vi "Acquire.vi"(6 "Count In":i32, 8 "error in (no error)":errorcluster, 9 "Data Queue":refnum<queue>, 10 "APD Data Notifier":refnum<notifier>, 11 "HW Resources In":T1={"Data Source"=0, "Counter Configuration"={"DAQmx Task"="", "Counter(s)"="Dev2/ctr0", "samples per readout"=100}, "ADC Configuration"={"DAQmx Task"="", "Channel(s)"="Dev2/ctr0", "samples per readout"=100, "Sample Rate (s/s)"=100, "Max Voltage"=100.0, "Min Voltage"=100.0}} {"Data Source" items=["Counter", "ADC"]}) -> (0 "error out":errorcluster, 3 "HW Resources Out":T1={"Data Source"=0, "Counter Configuration"={"DAQmx Task"="", "Counter(s)"="Dev2/ctr0", "samples per readout"=100}, "ADC Configuration"={"DAQmx Task"="", "Channel(s)"="Dev2/ctr0", "samples per readout"=100, "Sample Rate (s/s)"=100, "Max Voltage"=100.0, "Min Voltage"=100.0}} {"Data Source" items=["Counter", "ADC"]}, 4 "Cout Out":i32)   [LabVIEW 2013, in "Acquisition.lvlib"]
doc: "Perform the acquisition. Replace the contents of this diagram with calls to acquisition hardware."
uses:
  Acquisition.lvlib
  Hardware Configuration.ctl
  Counter Configuration.ctl
  ADC/ADC Configuration.ctl
  APD Notifier Cluster.ctl
  <vilib>/DAQmx/read.llb/DAQmx Read (Counter 1D DBL 1Chan NSamp).vi
  <vilib>/DAQmx/read.llb/DAQmx Read (Analog 1D Wfm NChan NSamp).vi
  <resource>/objmgr/daqmx.rc
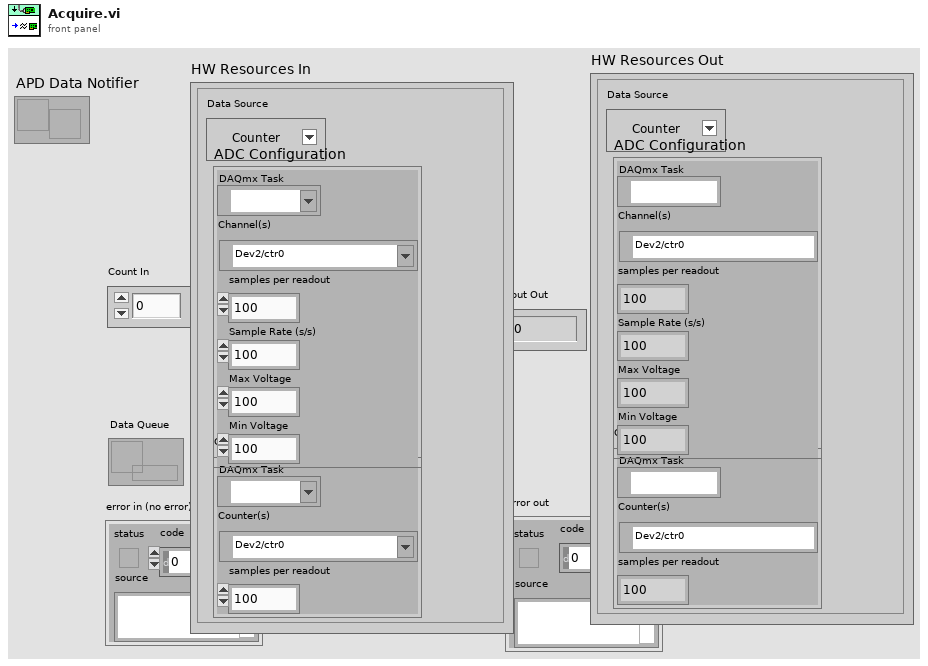
[diagram p1: front panel]
types:
  T1 = typedef "Acquisition.lvlib/Hardware Configuration.ctl" = cluster{"Data Source":u16, "Counter Configuration":T2, "ADC Configuration":T3}
  T2 = typedef "Acquisition.lvlib/Counter Configuration.ctl" = cluster{"DAQmx Task":refnum<k21>, "Counter(s)":tag, "samples per readout":i32}
  T3 = typedef "Acquisition.lvlib/ADC Configuration.ctl" = cluster{"DAQmx Task":refnum<k21>, "Channel(s)":tag, "samples per readout":i32, "Sample Rate (s/s)":i32, "Max Voltage":dbl, "Min Voltage":dbl}
  T4 = typedef "Acquisition.lvlib/APD Notifier Cluster.ctl" = cluster{"data":dbl[][], "t0":i32}
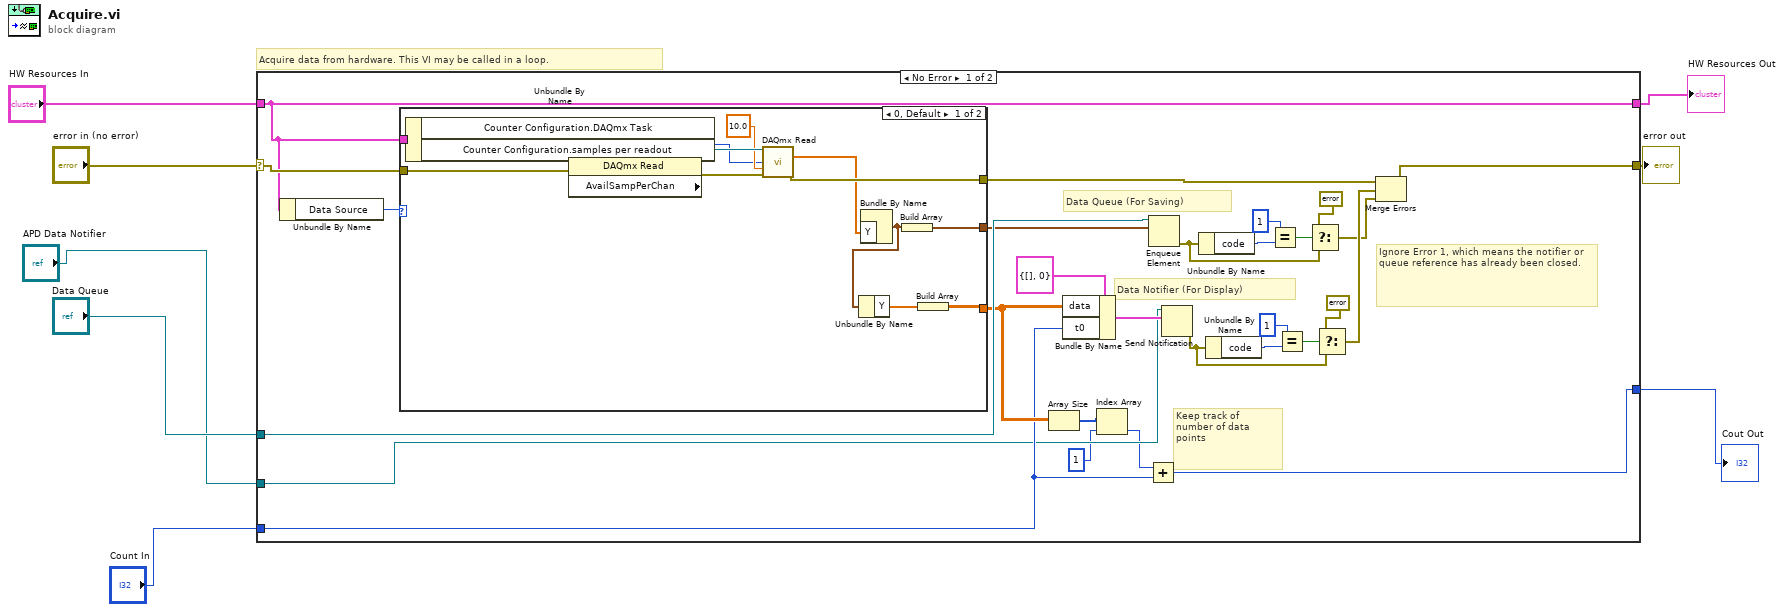
[diagram p0: block diagram]
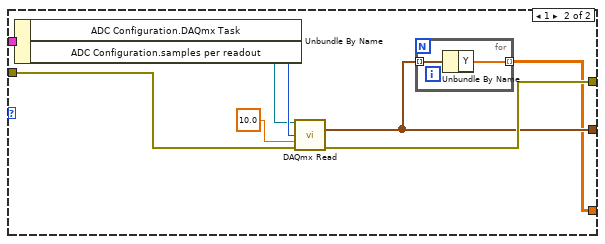
[diagram p2: hidden frame]
diagram:
  # "Acquire data from hardware. This VI may be called in a loop."
  n1 = case shown="No Error" "error in (no error)" {
    selector: "error in (no error)" -> [w22 w61]
    tunnel: [w36 w61] -> w7
    tunnel: "HW Resources In" -> [w14 w62]
    tunnel: [w14 w62] -> w3
    tunnel: "Data Queue" -> [w24 _]
    tunnel: "APD Data Notifier" -> [w12 _]
    tunnel: "Count In" -> [w15 w60]
    tunnel: [w19 w60] -> w4
    frame No Error {
      # "Data Notifier (For Display)"
      # "Data Queue (For Saving)"
      # "Keep track of\nnumber of data\npoints"
      # "Ignore Error 1, which means the notifier or queue reference has already been closed."
      n2 = Unbundle By Name(w14) -> ("Data Source"=w13:u16)
      n3 = case shown="0, Default" w13 {
        tunnel: w14 -> [w49 w57]
        tunnel: [w48 w56] -> w23
        tunnel: w22 -> [w46 w52]
        tunnel: [w41 w51] -> w21
        tunnel: [w39 w50] -> w16
        frame 0, Default {
          n4 = Unbundle By Name(w49) -> ("Counter Configuration.DAQmx Task"=w47:refnum<k21>, "Counter Configuration.samples per readout"=w43:i32)
          n5 = property class="DAQmx Read" props=["AvailSampPerChan"](reference=w47, error in=w46) -> (reference out=w45:refnum<k21>, error out=w42:errorcluster)  [unwired: 1 out]
          n6 = call-poly <vilib>:"DAQmx Read.vi"("task/channels in"=w45, "number of samples per channel"=w43, "timeout"=10.0, "error in"=w42) -> ("data"=w40:dbl[], "error out"=w48:errorcluster)  [unwired: 9 in, 1 out]
          n7 = Bundle By Name("Y"=w40) -> (w37:waveform(dbl))  [unwired: 1 in]
          n8 = Unbundle By Name(w37) -> ("Y"=w38:dbl[])
          n9 = Build Array(w37) -> (w41:waveform(dbl)[])
          n10 = Build Array(w38) -> (w39:dbl[][])
        }
        frame 1 {
          n11 = Unbundle By Name(w57) -> ("ADC Configuration.DAQmx Task"=w53:refnum<k21>, "ADC Configuration.samples per readout"=w54:i32)
          n12 = call-poly <vilib>:"DAQmx Read.vi"("task/channels in"=w53, "number of samples per channel"=w54, "timeout"=10.0, "error in"=w52) -> ("data"=w51:waveform(dbl)[], "error out"=w56:errorcluster)  [unwired: 9 in, 1 out]
          n13 = for {
            tunnel: w51 -> [w59] mode=indexing
            tunnel: [w58] -> w50 mode=indexing
            n14 = Unbundle By Name(w59) -> ("Y"=w58:dbl[])
          }
        }
      }
      n15 = Array Size(array=w16) -> (size(s)=w11:i32[])
      n16 = Bundle By Name(cluster=T4 {"data"=[], "t0"=0} ("APD Data Notifier Cluster"), "data"=w16, "t0"=w15) -> (w18:T4)
      n17 = Index Array(array=w11, index=1) -> (element=w9:i32)
      n18 = Add(x=w9, y=w15) -> (x+y=w19:i32)
      n19 = Enqueue Element(queue=w24, element=w21) -> (error out=w29:errorcluster)  [unwired: 2 in, 2 out]
      n20 = Send Notification(notification=w18, notifier=w12) -> (error out=w20:errorcluster)  [unwired: 1 in, 1 out]
      n21 = Unbundle By Name(w29) -> ("code"=w26:i32)
      n22 = Unbundle By Name(w20) -> ("code"=w35:i32)
      n23 = Equal?(x=1, y=w26) -> (x = y?=w28:bool)
      n24 = Equal?(x=1, y=w35) -> (x = y?=w33:bool)
      n25 = Select(t=errorcluster {"status"=FALSE, "code"=0, "source"=""} ("error constant"), s=w28, f=w29) -> (s? t:f=w25:errorcluster)
      n26 = Select(t=errorcluster {"status"=FALSE, "code"=0, "source"=""} ("error constant"), s=w33, f=w20) -> (s? t:f=w32:errorcluster)
      n27 = Merge Errors(w23, w32, w25) -> (w36:errorcluster)
    }
    frame Error {
    }
  }
  "error out" <- w7
  "Cout Out" <- w4
  "HW Resources Out" <- w3
